vi "Timing SubVI.vi"(6 "ID":string, 8 "Action":enum16{"Measure", "Report-n-Clear"}(ring), 9 "Image":T1, 10 "Boolean":bool, 11 "Numeric":dbl) -> (0 "Timings":cluster{u32, "ID":string}[](array[cluster]), 1 "Image 2":T1, 2 "Boolean 2":bool, 3 "Numeric 2":dbl)   [LabVIEW 2013]
uses:
  <vilib>/vision/Image Controls.llb/IMAQ Image.ctl
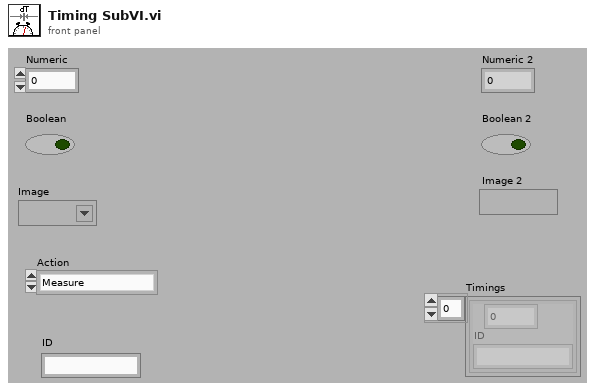
[diagram p1: front panel]
types:
  T1 = typedef "IMAQ Image.ctl" = refnum<image>
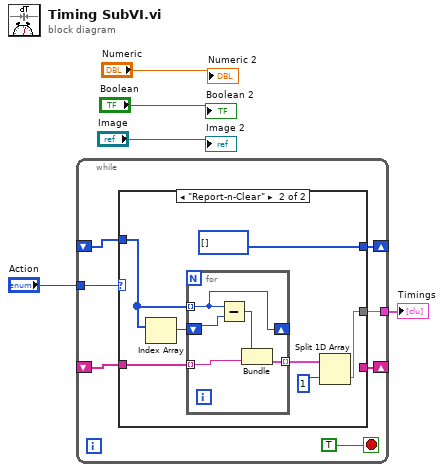
[diagram p0: block diagram]
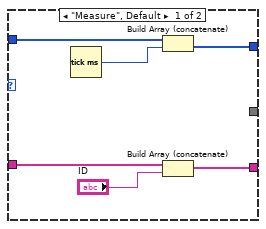
[diagram p2: hidden frame]
diagram:
  n1 = while {
    tunnel: "Action" -> [w12]
    shift-right: [w11] -> _
    shift-left: _ -> [w10]
    tunnel: [w8] -> w1
    shift-right: [w7] -> _
    shift-left: _ -> [w6]
    stop <- TRUE stop-if-true
    n2 = case shown="\"Report-n-Clear\"" w12 {
      tunnel: [w18 u32[] []] -> w11
      tunnel: w10 -> [w17 w24]
      tunnel: [_ w21] -> w8
      tunnel: [w15 _] -> w7
      tunnel: w6 -> [w14 w19]
      frame "Measure", Default {
        n3 = Tick Count (ms)() -> (millisecond timer value=w16:u32)
        n4 = Build Array (concatenate)(w17, w16) -> (w18:u32[])
        n5 = Build Array (concatenate)(w14, "ID") -> (w15:string[])
      }
      frame "Report-n-Clear" {
        n6 = Index Array(array=w24) -> (element=w23:u32)  [unwired: 1 in]
        n7 = for {
          tunnel: w24 -> [w29] mode=indexing
          shift-right: [w29] -> _
          shift-left: w23 -> [w30]
          tunnel: [w27] -> w22 mode=indexing
          tunnel: w19 -> [w26] mode=indexing
          n8 = Subtract(x=w29, y=w30) -> (x-y=w28:u32)
          n9 = Bundle(w28, "ID"=w26) -> (w27:cluster{u32, "ID":string})  [unwired: 1 in]
        }
        n10 = Split 1D Array(array=w22, index=1) -> (second subarray=w21:cluster{u32, "ID":string}[])  [unwired: 1 out]
      }
    }
  }
  "Timings" <- w1
  "Numeric 2" <- "Numeric"
  "Boolean 2" <- "Boolean"
  "Image 2" <- "Image"
